vi "Koheras.vi"(10 "error in (no error)":errorcluster) -> ()   [LabVIEW 2011]
uses:
  Utilities/controls/ctlSeqFNs_PCDeviceInit.ctl
  Utilities/controls/ctlSeqFNs_Main.ctl
  Utilities/controls/ctlSeqFNs_Koheras.ctl
  <vilib>/userDefined/High Color/IMAQdx.ctl
panel:
  out "out":errorcluster
  in  "error in":errorcluster
  out "error out":errorcluster
  in  "config remote device":T2
  in  "remote device online status":T3
  in  "KoherasSet":string[](array[string])
  in  "terminal out":T4
  in  "interface management remote device":T5
  in  "set remote device online":T3
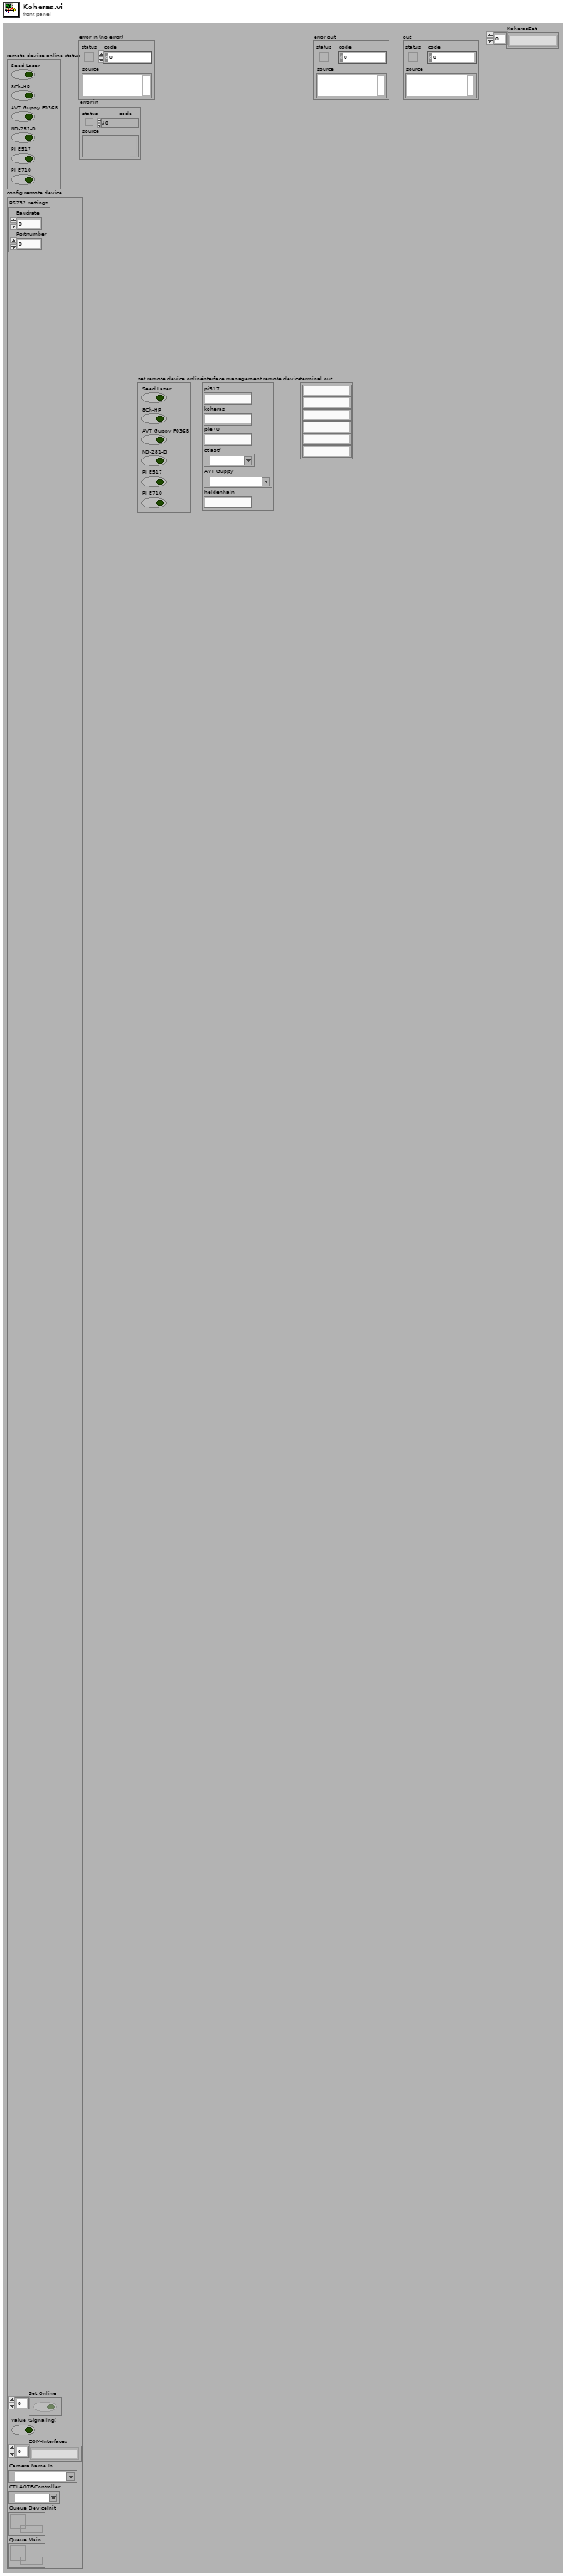
[diagram p1: front panel]
types:
  T1 = typedef "IMAQdx.ctl" = refnum<k21>
  T2 = cluster{"RS232 settings":cluster{"Baudrate":u16, "Portnumber":i32}, "Set Online":bool[], "Value (Signaling)":bool, "COM-Interfaces":string[], "Camera Name In":T1, "CTI AOTF-Controller":refnum<visa-resource-name>, "Queue DeviceInit":refnum<queue>, "Queue Main":refnum<queue>}
  T3 = cluster{"Seed Laser":bool, "8Ch-HP":bool, "AVT Guppy F036B":bool, "ND-281-D":bool, "PI E517":bool, "PI E710":bool}
  T4 = cluster{string, string, string, string, string, string}
  T5 = cluster{"pi517":string, "koheras":string, "pie70":string, "ctiaotf":refnum<visa-resource-name>, "AVT Guppy":T1, "heidenhain":string}
  T6 = typedef "ctlSeqFNs_Koheras.ctl" = enum16{"ERROR", "INIT", "Initialization", "Configuration", "Measurement", "Shutdown", "IDLE", "EXIT"}
  T7 = cluster{"Queue Main":refnum<queue>, "Queue DeviceInit":refnum<queue>, "set remote device online":cluster{"Seed Laser":bool, "8Ch-HP":bool, "AVT Guppy F036B":bool, "ND-281-D":bool, "PI E517":bool, "PI E710":bool}, "config remote device":cluster{"RS232 settings":cluster{"Baudrate":u16, "Portnumber":i32}, "Set Online":bool[], "Value (Signaling)":bool, "COM-Interfaces":string[], "Camera Name In":T1, "CTI AOTF-Controller":refnum<visa-resource-name>, "Queue DeviceInit":refnum<queue>, "Queue Main":refnum<queue>}, "remote device online status":cluster{"Seed Laser":bool, "8Ch-HP":bool, "AVT Guppy F036B":bool, "ND-281-D":bool, "PI E517":bool, "PI E710":bool}, "interface management remote device":cluster{"pi517":string, "koheras":string, "pie70":string, "ctiaotf":refnum<visa-resource-name>, "AVT Guppy":T1, "heidenhain":string}, "terminal out":cluster{string, string, string, string, string, string}, "KoherasSet":string[]}
  T8 = typedef "ctlSeqFNs_Main.ctl" = enum16{"ERROR", "INIT", "CONFIGURE", "MEASUREMENT", "SHUTDOWN", "IDLE", "EXIT"}
  T9 = typedef "ctlSeqFNs_PCDeviceInit.ctl" = enum16{"ERROR", "INIT", "ErrorDevice", "StartDevice", "DeviceStatus", "StopDevice", "EXIT", "IDLE"}
  T10 = cluster{"Seed Laser Power 2":i8, "LaserPowerConfigure 2":bool}
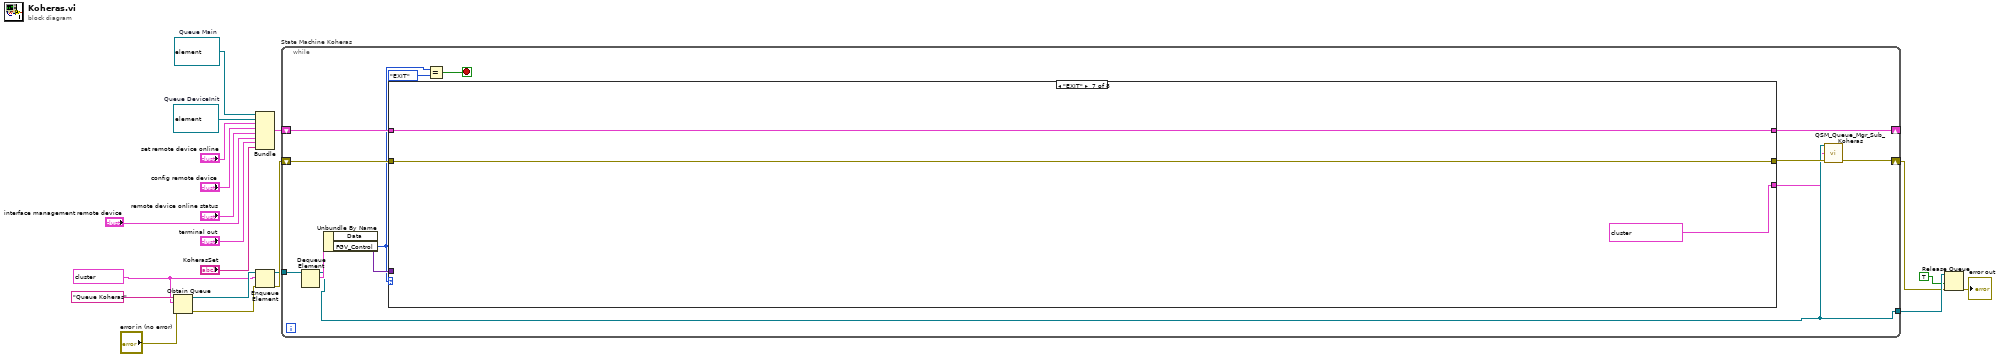
[diagram p0: block diagram]
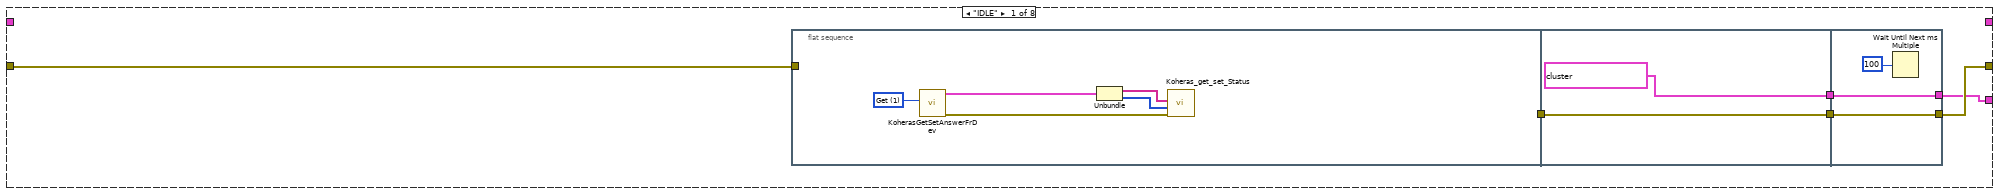
[diagram p2: hidden frame]
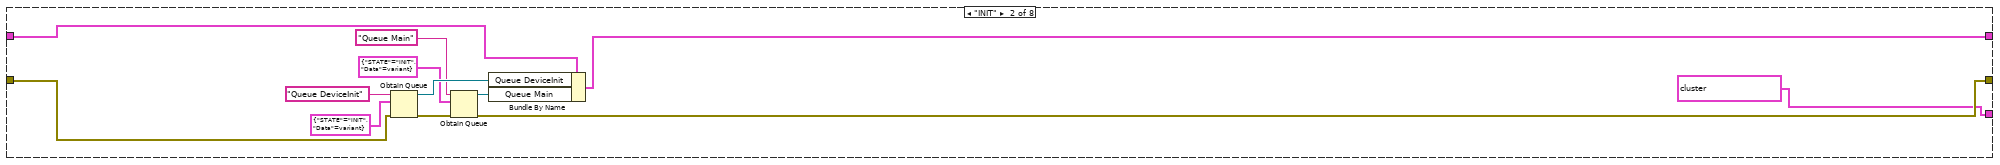
[diagram p3: hidden frame]
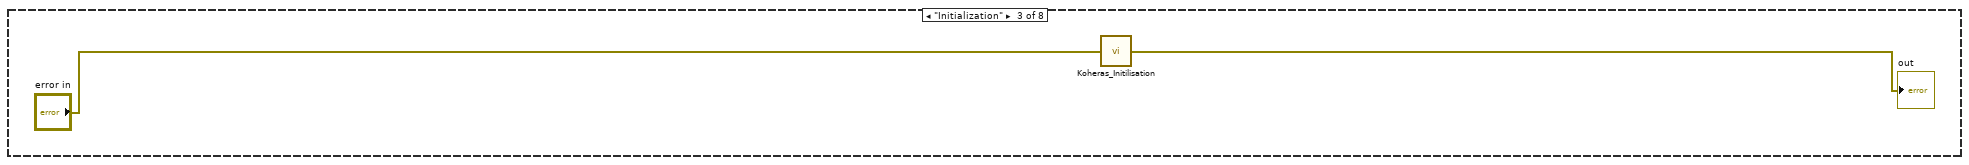
[diagram p4: hidden frame]
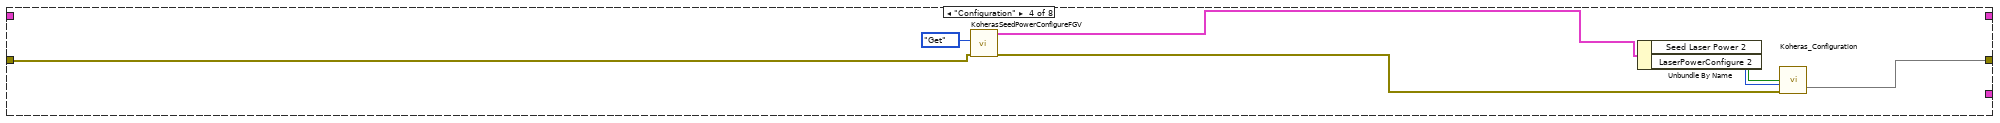
[diagram p5: hidden frame]
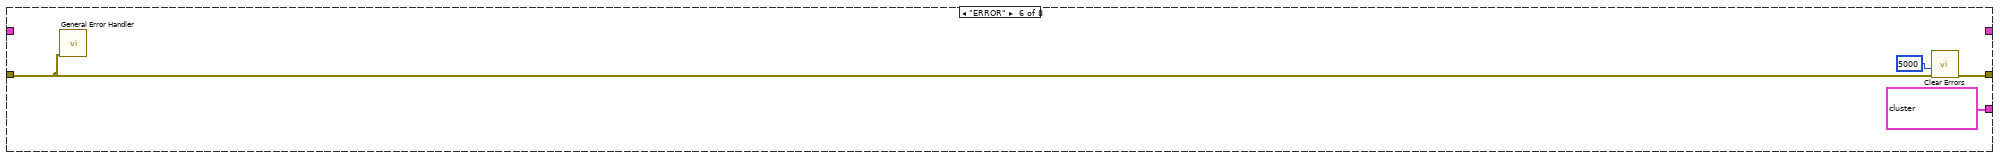
[diagram p7: hidden frame]
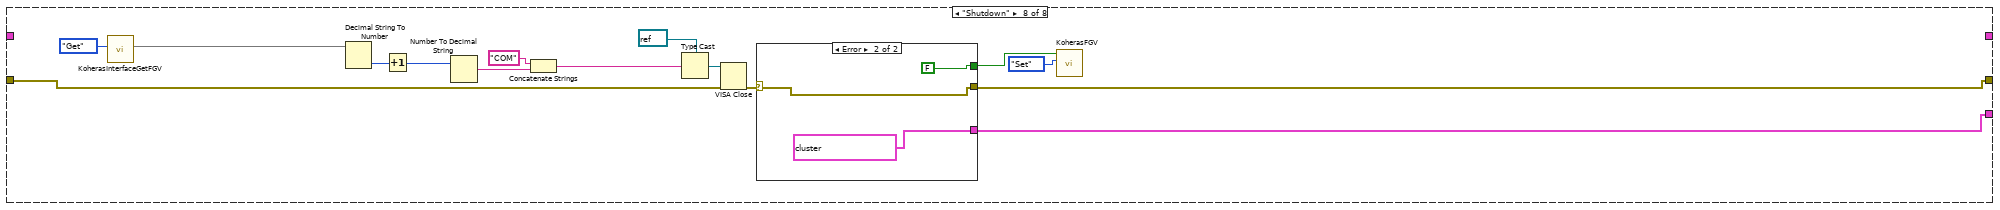
[diagram p8: hidden frame]
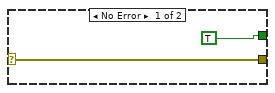
[diagram p9: hidden frame]
diagram:
  w2 = cluster{"Data":variant, "FGV_Control":T6} {"Data"=variant, "FGV_Control"=enum."ERROR"} ("element")
  w9 = refnum<queue> refnum  # Queue Main
  w8 = refnum<queue> refnum  # Queue DeviceInit
  n1 = Obtain Queue(name (unnamed)="Queue Koheras", element data type=w2, error in (no error)="error in (no error)") -> (queue out=w17:refnum<queue>, error out=w19:errorcluster)  [unwired: 2 in, 1 out]
  n2 = Bundle("Queue Main"=w9, "Queue DeviceInit"=w8, "set remote device online"="set remote device online", "config remote device"="config remote device", "remote device online status"="remote device online status", "interface management remote device"="interface management remote device", "terminal out"="terminal out", "KoherasSet"="KoherasSet") -> (w16:T7)  [unwired: 1 in]
  n3 = Enqueue Element(queue=w17, element=w2, error in (no error)=w19) -> (queue out=w15:refnum<queue>, error out=w18:errorcluster)  [unwired: 1 in, 1 out]
  n4 = while "State Machine Koheras" {
    shift-right: [w24] -> w5
    shift-left: w18 -> [w33]
    tunnel: w15 -> [w23]
    tunnel: [w22] -> w6
    shift-right: [w28] -> _
    shift-left: w16 -> [w29]
    stop <- w32 stop-if-true
    n5 = Dequeue Element(queue=w23) -> (queue out=w22:refnum<queue>, element=w31:cluster{"Data":variant, "FGV_Control":T6})  [unwired: 2 in, 2 out]
    n6 = Unbundle By Name(w31) -> ("Data"=w30:variant, "FGV_Control"=w27:T6)
    n7 = case shown="\"EXIT\"" w27 {
      tunnel: w33 -> [w36 w57 _ w69 w71 w75 w79 w94]
      tunnel: w30 -> [_ _ _ _ _ _ _ _]
      tunnel: w29 -> [_ w60 _ _ w72 _ w78 _]
      tunnel: [_ w59 _ _ w72 _ w78 _] -> w28
      tunnel: [w37 w52 _ w70 w71 w74 w79 w92] -> w25
      tunnel: [w34 cluster{"Data":variant, "FGV_Control":T6}[] [{"Data"=variant, "FGV_Control"=enum."IDLE"}] ("QSTATES") _ _ _ cluster{"Data":variant, "FGV_Control":T6}[] [{"Data"=variant, "FGV_Control"=enum."IDLE"}] ("QSTATES") cluster{"Data":variant, "FGV_Control":T6}[] [{"Data"=variant, "FGV_Control"=enum."EXIT"}] ("QSTATES") w80] -> w21
      frame "IDLE" {
        n8 = flat-sequence {
          tunnel: w36 -> [_]
          tunnel: [_] -> w39
          tunnel: w39 -> [w46]
          tunnel: [w46] -> w38
          tunnel: [cluster{"Data":variant, "FGV_Control":T6}[] [{"Data"=variant, "FGV_Control"=enum."IDLE"}] ("QSTATES")] -> w35
          tunnel: w38 -> [w48]
          tunnel: [w48] -> w37
          tunnel: [w47] -> w34
          tunnel: w35 -> [w47]
          frame #0 {
            w43 = u16 1 items=["Set", "Get"] ("FGV_Control")
            n9 = call "KoherasGetSetAnswerFrDev.vi"("FGV_Control"=w43) -> ("error out"=w44:errorcluster, "out"=w42:cluster{string[], i32[]})  [unwired: 9 in]
            n10 = Unbundle(w42) -> (w41:string[], w40:i32[])
            n11 = call "Koheras_get_set_Status.vi"("error in"=w44, "Array 2"=w40, "Array"=w41) -> ()  [unwired: 6 in, 3 out]
          }
          frame #1 {
          }
          frame #2 {
            n12 = Wait Until Next ms Multiple(millisecond multiple=u32 100) -> ()  [unwired: 1 out]
          }
        }
      }
      frame "INIT" {
        n13 = Obtain Queue(name (unnamed)="Queue DeviceInit" ("Queue Name"), element data type=cluster{"STATE":T9, "Data":variant} {"STATE"=enum."INIT", "Data"=variant} ("element"), error in (no error)=w57) -> (queue out=w58:refnum<queue>, error out=w53:errorcluster)  [unwired: 2 in, 1 out]
        n14 = Obtain Queue(name (unnamed)="Queue Main" ("Queue Name"), element data type=cluster{"STATE":T8, "Data":variant} {"STATE"=enum."INIT", "Data"=variant} ("element"), error in (no error)=w53) -> (queue out=w51:refnum<queue>, error out=w52:errorcluster)  [unwired: 2 in, 1 out]
        n15 = Bundle By Name(cluster=w60, "Queue DeviceInit"=w58, "Queue Main"=w51) -> (w59:T7)
      }
      frame "Initialization" {
        n16 = call "Koheras_Initilisation.vi"("error in"="error in") -> ("error out"=→"out":errorcluster)
      }
      frame "Configuration" {
        n17 = call "KoherasSeedPowerConfigureFGV.vi"("error in"=w69, "Set_Get"=enum16{"Set", "Get"}."Get") -> ("error out"=w66:errorcluster, "SeedLaserPower"=w67:T10)  [unwired: 8 in]
        n18 = Unbundle By Name(w67) -> ("Seed Laser Power 2"=w65:i8, "LaserPowerConfigure 2"=w64:bool)
        n19 = call "Koheras_Configuration.vi"(2:w65, 3:w66, 4:w64) -> (6:w70)  [unwired: 3 in]
      }
      frame "Measurement" {
      }
      frame "ERROR" {
        n20 = call <vilib>:"General Error Handler.vi"("error in (no error)"=w75) -> ()  [unwired: 10 in, 5 out]
        n21 = call <vilib>:"Clear Errors.vi"("error in (no error)"=w75, 5:u32 5000 ("wait(ms)")) -> ("error out"=w74:errorcluster)  [unwired: 5 in]
      }
      frame "EXIT" {
      }
      frame "Shutdown" {
        n22 = call "KoherasInterfaceGetFGV.vi"("Set_Get"=enum16{"Set", "Get"}."Get") -> (2:w82)  [unwired: 8 in, 2 out]
        n23 = Decimal String To Number(string=w82) -> (number=w85:i32)  [unwired: 2 in, 1 out]
        n24 = Increment(x=w85) -> (x+1=w84:i32)
        n25 = Number To Decimal String(number=w84) -> (decimal integer string=w83:string)  [unwired: 1 in]
        n26 = Concatenate Strings("COM" ("string"), w83) -> (w86:string)
        n27 = Type Cast(type=refnum<visa-resource-name> refnum ("VISA resource name"), x=w86) -> (*(type *) &x=w81:refnum<visa-resource-name>)
        n28 = VISA Close(VISA resource name=w81, error in (no error)=w94) -> (error out=w93:errorcluster)
        n29 = case shown="Error" w93 {
          selector: w93 -> [w96 w99]
          tunnel: [w96 w99] -> w92
          tunnel: [TRUE ("KoherasLaser") FALSE ("KoherasLaser")] -> w91
          tunnel: [_ cluster{"Data":variant, "FGV_Control":T6}[] [{"Data"=variant, "FGV_Control"=enum."ERROR"}] ("QSTATES")] -> w80
          frame No Error {
          }
          frame Error {
          }
        }
        n30 = call "KoherasFGV.vi"("Set_Get"=enum16{"Set", "Get"}."Set", "Value"=w91) -> ()  [unwired: 8 in, 2 out]
      }
    }
    n31 = Equal?(x=w27, y=ctlSeqFNs_Koheras."EXIT" ("FGV_Control 2")) -> (x = y?=w32:bool)
    n32 = call "QSM_Queue_Mgr_Sub_Koheras.vi"("queue out"=w22, "QSTATES"=w21, "Error IN 2"=w25) -> ("Error OUT 2"=w24:errorcluster)  [unwired: 12 in]
  }
  n33 = Release Queue(queue=w6, force destroy? (F)=TRUE, error in (no error)=w5) -> (error out=→"error out":errorcluster)  [unwired: 2 out]
